vi "TempsÉcouléGen.vi"(8 "error in (no error)":errorcluster caption="entrée d'erreur", 9 "Points effectués":i32, 10 "Points restant":u32, 11 "Temps initiale":u32) -> (0 "error out":errorcluster caption="sortie d'erreur", 1 "Temps Restant":dbl, 2 "Temps Écoulé":u32, 3 "Temps Actuel":u32)   [LabVIEW 2012]
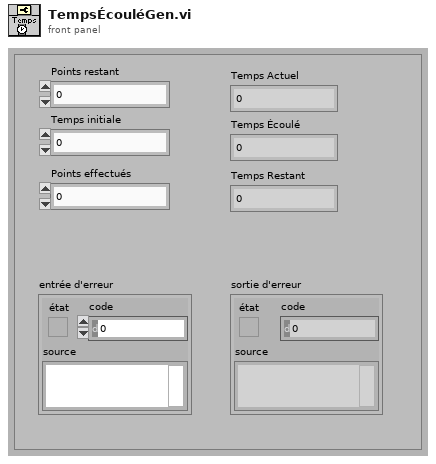
[diagram p1: front panel]
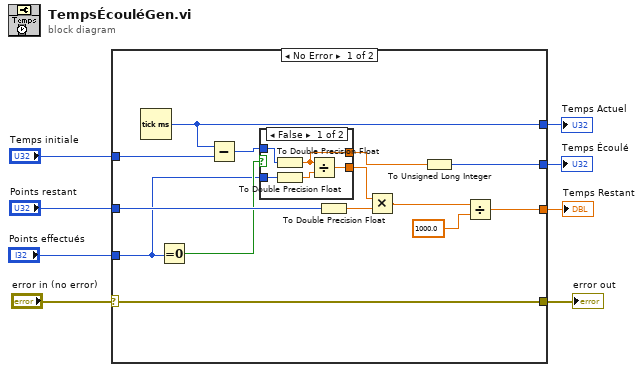
[diagram p0: block diagram]
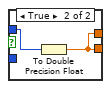
[diagram p2: hidden frame]
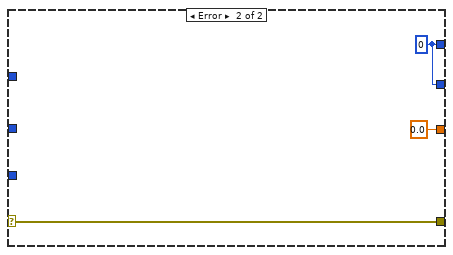
[diagram p3: hidden frame]
diagram:
  n1 = case shown="No Error" "error in (no error)" {
    selector: "error in (no error)" -> [w22 w32]
    tunnel: "Temps initiale" -> [w21 _]
    tunnel: [w22 w32] -> w6
    tunnel: [w20 w30] -> w5
    tunnel: "Points restant" -> [w19 _]
    tunnel: [w17 0.0] -> w3
    tunnel: [w10 w30] -> w2
    tunnel: "Points effectués" -> [w13 _]
    frame No Error {
      n2 = Tick Count (ms)() -> (millisecond timer value=w20:u32)
      n3 = Equal To 0?(x=w13) -> (x = 0?=w16:bool)
      n4 = Subtract(x=w20, y=w21) -> (x-y=w14:u32)
      n5 = case shown="False" w16 {
        tunnel: [w26 w28] -> w15
        tunnel: w14 -> [w27 w29]
        tunnel: w13 -> [w25 _]
        tunnel: [w23 w28] -> w9
        frame False {
          n6 = To Double Precision Float(number=w27) -> (double precision float=w23:dbl)
          n7 = To Double Precision Float(number=w25) -> (double precision float=w24:dbl)
          n8 = Divide(x=w23, y=w24) -> (x/y=w26:dbl)
        }
        frame True {
          n9 = To Double Precision Float(number=w29) -> (double precision float=w28:dbl)
        }
      }
      n10 = To Double Precision Float(number=w19) -> (double precision float=w12:dbl)
      n11 = Multiply(x=w15, y=w12) -> (x*y=w11:dbl)
      n12 = To Unsigned Long Integer(number=w9) -> (unsigned 32bit integer=w10:u32)
      n13 = Divide(x=w11, y=1000.0) -> (x/y=w17:dbl)
    }
    frame Error {
      w30 = u32 0 ("millisecond timer value")
    }
  }
  "error out" <- w6
  "Temps Actuel" <- w5
  "Temps Restant" <- w3
  "Temps Écoulé" <- w2
